vi "Initialise.vi"(8 "error in (no error)":errorcluster, 10 "Message in":refnum<class "InitialiseMessage.lvclass">, 11 "AOTF in":refnum<class "AOTF.lvclass">) -> (0 "error out":errorcluster, 3 "AOTF out":refnum<class "AOTF.lvclass">)   [LabVIEW 2012, in "AOTF.lvclass"]
doc: "This method is called when an initialise message is received. It mainly initialises the RabbitMQ connectivity. \n\nOverride this method when your component needs special initialisation (e.g. of software or hardware resources). In that case, don't forget to call the parent for proper implementation. If your component owns subcomponents, they count as resources, so you have to initialise them by calling their own initialise functions"
uses:
  AOTF.lvclass
  <vilib>/Distrio/Murmex/InitialiseMessage/InitialiseMessage.lvclass
  <vilib>/Distrio/Murmex/Murmex/Murmex.lvclass
  AOTF.lvclass/AOTF.ctl
  <vilib>/DAQmx/create/channels.llb/DAQmx Create Channel (DO-Digital Output).vi
  <vilib>/DAQmx/create/channels.llb/DAQmx Create Channel (AO-Voltage-Basic).vi
panel:
  # "This method is called when the INTIALISE\ntrigger is sent. \n\nOverride this method when your component needs to\nrespond to this trigger. \n\nCall parent for proper implementation"
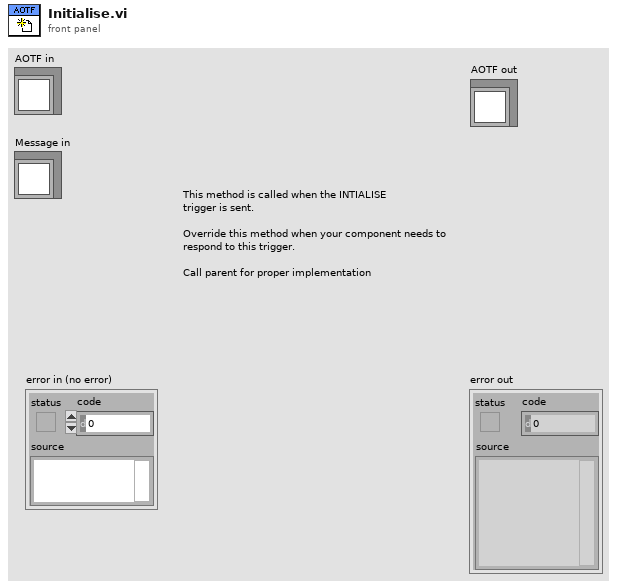
[diagram p1: front panel]
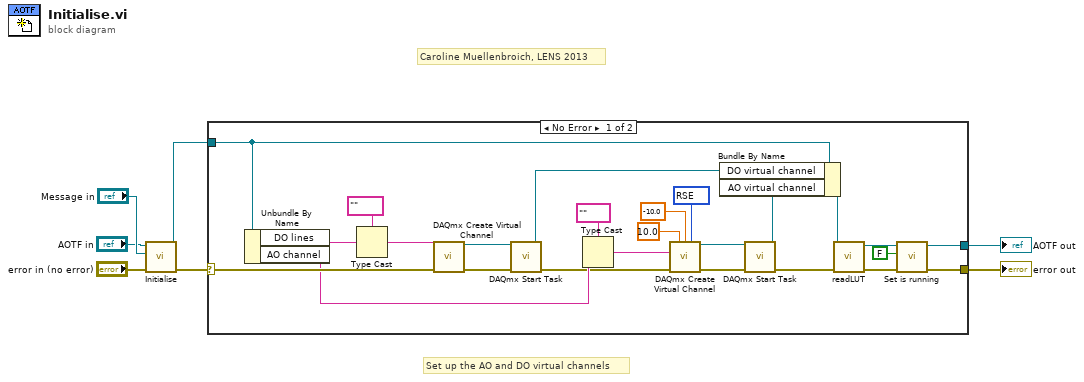
[diagram p0: block diagram]
diagram:
  # "Set up the AO and DO virtual channels"
  # "Caroline Muellenbroich, LENS 2013"
  n1 = call-parent "Initialise.vi"("error in (no error)"="error in (no error)", "Message in"="Message in", "Murmex in"="AOTF in") -> ("error out"=w4:errorcluster, "Murmex out"=w3:refnum<class "AOTF.lvclass">)  [unwired: 7 in]
  n2 = case shown="No Error" w4 {
    selector: w4 -> [w29 w34]
    tunnel: w3 -> [w30 w33]
    tunnel: [w11 w34] -> w2
    tunnel: [w9 w33] -> w1
    frame No Error {
      w28 = 10083 items=["Default"=-1, "RSE"=10083, "Differential"=10106, "Pseudodifferential"=12529] ("output terminal configuration")
      n3 = Unbundle By Name(w30) -> ("DO lines"=w21:string, "AO channel"=w16:string)
      n4 = Type Cast(type=tag "" ("lines"), x=w21) -> (*(type *) &x=w19:tag)
      n5 = call-poly <vilib>:"DAQmx Create Virtual Channel.vi"("lines"=w19, "error in"=w29) -> ("task out"=w24:refnum<k21>, "error out"=w25:errorcluster)  [unwired: 12 in]
      n6 = call <vilib>:"DAQmx Start Task.vi"("task/channels in"=w24, "error in"=w25) -> ("task out"=w14:refnum<k21>, "error out"=w15:errorcluster)  [unwired: 12 in]
      n7 = Type Cast(type=tag "" ("physical channels"), x=w16) -> (*(type *) &x=w17:tag)
      n8 = call-poly <vilib>:"DAQmx Create Virtual Channel.vi"("maximum value"=10.0, "minimum value"=-10.0, "output terminal configuration"=w28, "physical channels"=w17, "error in"=w15) -> ("task out"=w22:refnum<k21>, "error out"=w23:errorcluster)  [unwired: 9 in]
      n9 = call <vilib>:"DAQmx Start Task.vi"("task/channels in"=w22, "error in"=w23) -> ("task out"=w13:refnum<k21>, "error out"=w12:errorcluster)  [unwired: 12 in]
      n10 = Bundle By Name(cluster=w30, "DO virtual channel"=w14, "AO virtual channel"=w13) -> (w31:refnum<class "AOTF.lvclass">)
      n11 = call-dynamic "readLUT.vi"("error in (no error)"=w12, "AOTF in"=w31) -> ("error out"=w32:errorcluster, "AOTF out"=w10:refnum<class "AOTF.lvclass">)  [unwired: 8 in]
      n12 = call-dynamic "Set is running.vi"("error in (no error)"=w32, "is running?"=FALSE, "AOTF in"=w10) -> ("error out"=w11:errorcluster, "AOTF out"=w9:refnum<class "AOTF.lvclass">)  [unwired: 7 in]
    }
    frame Error {
    }
  }
  "error out" <- w2
  "AOTF out" <- w1
